vi "Read DC value.vi"(8 "error in (no error)":errorcluster, 11 "LHW-WfmBasicProperties in":refnum<class "LHW-WfmBasicProperties.lvclass">) -> (0 "error out":errorcluster, 2 "DC value":dbl[unit] format="%0.2p", 3 "LHW-WfmBasicProperties out":refnum<class "LHW-WfmBasicProperties.lvclass">)   [LabVIEW 2014, in "LHW-Data.lvlib" / "LHW-WfmBasicProperties.lvclass"]
uses:
  LHW-WfmBasicProperties.lvclass
  LHW-WfmBasicProperties.lvclass/LHW-WfmBasicProperties.ctl
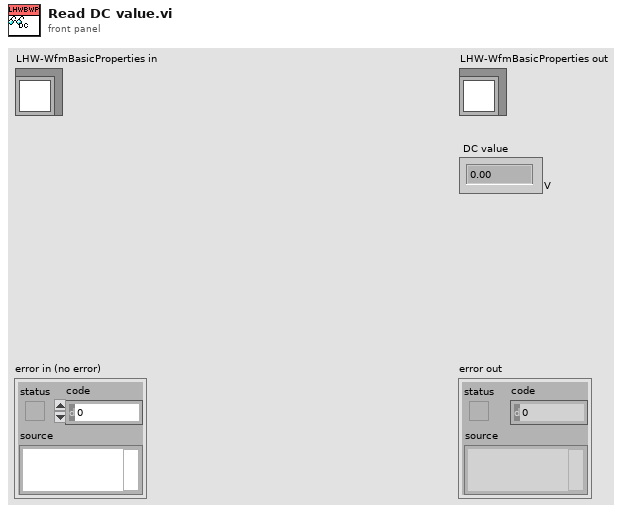
[diagram p1: front panel]
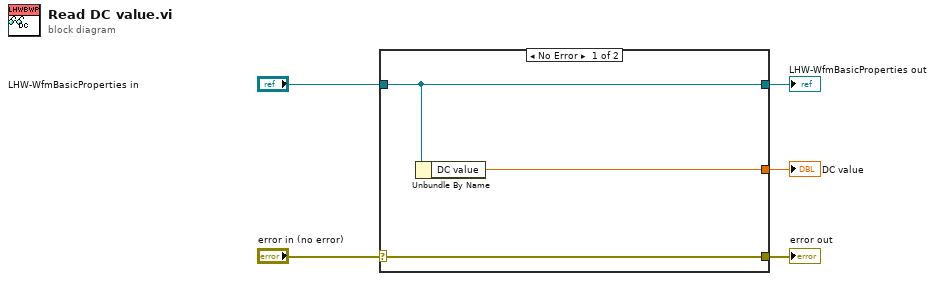
[diagram p0: block diagram]
diagram:
  n1 = case shown="No Error" "error in (no error)" {
    selector: "error in (no error)" -> [w8 w9]
    tunnel: [w8 w9] -> w4
    tunnel: [w7 w10] -> w2
    tunnel: "LHW-WfmBasicProperties in" -> [w7 w10]
    tunnel: [w6 _] -> w1
    frame No Error {
      n2 = Unbundle By Name(w7) -> ("DC value"=w6:dbl[unit])
    }
    frame Error {
    }
  }
  "error out" <- w4
  "LHW-WfmBasicProperties out" <- w2
  "DC value" <- w1
